vi "Read Aux.vi"(11 "JoystickDevRef":T1={"Device"=enum."USB 1"}) -> ()   [LabVIEW 2018]
uses:
  <vilib>/Rock Robotics/WPI/Joystick/WPI_JoystickDevRef.ctl
  <vilib>/Rock Robotics/WPI/Joystick/WPI_JoystickDeviceEnum.ctl
  Robot Global Data.vi
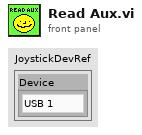
[diagram p1: front panel]
types:
  T1 = typedef "WPI_JoystickDevRef.ctl" = cluster{"Device":T2}
  T2 = typedef "WPI_JoystickDeviceEnum.ctl" = enum16{"USB 0", "USB 1", "USB 2", "USB 3", "USB 4", "USB 5"}
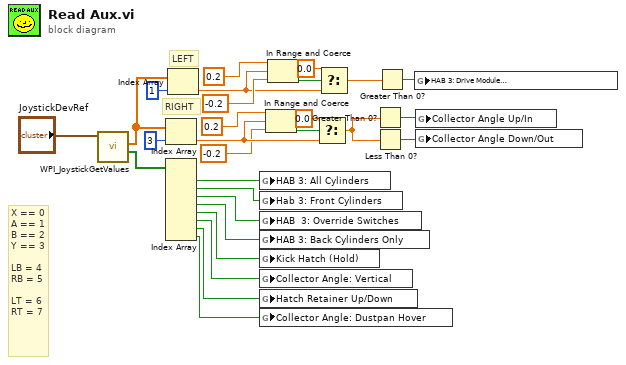
[diagram p0: block diagram]
diagram:
  # "LEFT"
  # "RIGHT"
  # "X == 0\nA == 1\nB == 2\nY == 3\n\nLB = 4\nRB = 5\n\nLT = 6\nRT = 7"
  n1 = call <vilib>:"WPI_JoystickGetValues.vi"("JoystickDevRef"="JoystickDevRef") -> ("Buttons"=w27:bool[], "Axes"=w9:dbl[])  [unwired: 6 in, 3 out]
  n2 = Index Array(array=w9, index=3) -> (element=w16:dbl)
  n3 = Index Array(array=w27) -> (element #1=w25:bool, element #2=w24:bool, element #3=w23:bool, element #4=w22:bool, element #5=w21:bool, element #6=w20:bool, element #7=w19:bool, element #8=w18:bool)  [unwired: 8 in]
  n4 = Index Array(array=w9, index=1) -> (element=w1:dbl)
  n5 = global write "Robot Global Data.vi" "HAB 3: All Cylinders"(w25) -> ()
  n6 = global write "Robot Global Data.vi" "Hab 3: Front Cylinders"(w24) -> ()
  n7 = global write "Robot Global Data.vi" "HAB  3: Override Switches"(w23) -> ()
  n8 = global write "Robot Global Data.vi" "HAB 3: Back Cylinders Only"(w22) -> ()
  n9 = global write "Robot Global Data.vi" "Kick Hatch (Hold)"(w21) -> ()
  n10 = global write "Robot Global Data.vi" "Collector Angle: Vertical"(w20) -> ()
  n11 = global write "Robot Global Data.vi" "Hatch Retainer Up/Down"(w19) -> ()
  n12 = global write "Robot Global Data.vi" "Collector Angle: Dustpan Hover"(w18) -> ()
  n13 = In Range and Coerce(upper limit=0.2, x=w16, lower limit=-0.2) -> (In Range?=w17:bool)  [unwired: 1 out]
  n14 = In Range and Coerce(upper limit=0.2, x=w1, lower limit=-0.2) -> (In Range?=w7:bool)  [unwired: 1 out]
  n15 = Select(t=0.0, s=w17, f=w16) -> (s? t:f=w12:dbl)
  n16 = Select(t=0.0, s=w7, f=w1) -> (s? t:f=w3:dbl)
  n17 = Greater Than 0?(x=w12) -> (x > 0?=w11:bool)
  n18 = Less Than 0?(x=w12) -> (x < 0?=w10:bool)
  n19 = Greater Than 0?(x=w3) -> (x > 0?=w2:bool)
  n20 = global write "Robot Global Data.vi" "HAB 3: Drive Module\n(FORWARD)"(w2) -> ()
  n21 = global write "Robot Global Data.vi" "Collector Angle Up/In"(w11) -> ()
  n22 = global write "Robot Global Data.vi" "Collector Angle Down/Out"(w10) -> ()
